vi "Get DI DAQ SMQ - single.vi"(8 "error in (no error)":errorcluster, 9 "AI TaskName":string, 10 "AI Thread SMQs":variant) -> (0 "error out":errorcluster, 1 "AI DAQ SMQ":refnum<queue>, 2 "AI Thread SMQs out":variant)   [LabVIEW 2017, in "DAQ.lvclass"]
doc: "Developed by Kevin Thompson\nkevin@thompsonengineering.net\n\nCopyright 2018-2020\nThompson Engineering, LLC"
uses:
  DAQ.lvclass
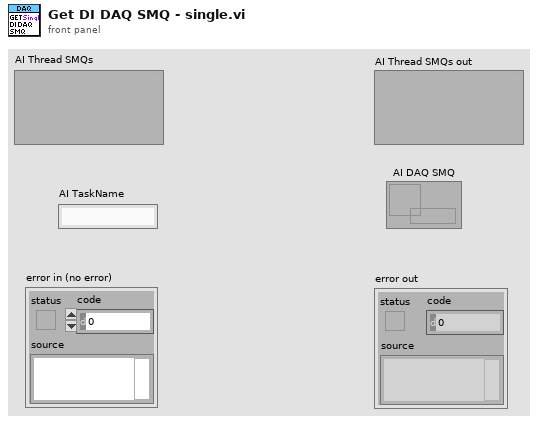
[diagram p1: front panel]
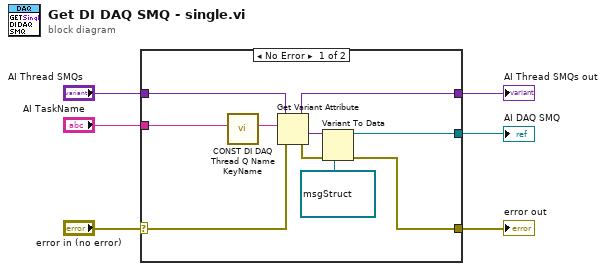
[diagram p0: block diagram]
diagram:
  n1 = case shown="No Error" "error in (no error)" {
    selector: "error in (no error)" -> [w11 w18]
    tunnel: [w10 w18] -> w5
    tunnel: "AI TaskName" -> [w13 _]
    tunnel: "AI Thread SMQs" -> [w9 w17]
    tunnel: [w8 _] -> w2
    tunnel: [w7 w17] -> w1
    frame No Error {
      n2 = call "CONST DI DAQ Thread Q Name KeyName.vi"("DI TaskName"=w13) -> ("DI SMQ (KeyName)"=w14:string)  [unwired: 10 in]
      n3 = Get Variant Attribute(Variant=w9, name=w14, error in=w11) -> (duplicate Variant=w7:variant, value=w15:variant, error out=w12:errorcluster)  [unwired: 1 in, 1 out]
      n4 = Variant To Data(error in=w12, type=refnum<queue> refnum ("AI DAQ SMQ"), Variant=w15) -> (data=w8:refnum<queue>, error out=w10:errorcluster)
    }
    frame Error {
    }
  }
  "error out" <- w5
  "AI DAQ SMQ" <- w2
  "AI Thread SMQs out" <- w1
